vi "Config 135 via GPIB.vi"(3 "error in":T1, 4 "Configuration (in)":T3={"Sensor Length (cm)"=100.0, "Hi Setpoint (cm)"=80.0, "Lo Setpoint (cm)"=20.0, "Sampling Interval (min)"=1.0} {"Sampling Interval (min)" min=0 max=600 format="%.1f"; "Lo Setpoint (cm)" min=0 max=203.2 format="%.1f"; "Hi Setpoint (cm)" min=0 max=203.2 format="%.1f"; "Sensor Length (cm)" min=1 max=203.2 format="%.1f"}, 5 "Hidden Controls (in)":T2 {"Prev Sampling Interval" format="%.1f"; "Prev Lo Setpoint" format="%.1f"; "Prev Hi Setpoint" format="%.1f"; "Prev Sensor Length" format="%.1f"; "Helium Level (cm)" format="%.1f"}, 6 "GPIB Setup":cluster{"GPIB address":i16, "GPIB bus":i16}={"GPIB address"=1, "GPIB bus"=0}) -> (0 "error out":T1, 1 "Hidden Controls (out)":T2 {"Prev Sampling Interval" format="%.1f"; "Prev Lo Setpoint" format="%.1f"; "Prev Hi Setpoint" format="%.1f"; "Prev Sensor Length" format="%.1f"; "Helium Level (cm)" format="%.1f"}, 2 "Configuration (out)":T3={"Sensor Length (cm)"=100.0, "Hi Setpoint (cm)"=80.0, "Lo Setpoint (cm)"=20.0, "Sampling Interval (min)"=1.0} {"Sampling Interval (min)" min=0 max=600 format="%.1f"; "Lo Setpoint (cm)" min=0 max=203.2 format="%.1f"; "Hi Setpoint (cm)" min=0 max=203.2 format="%.1f"; "Sensor Length (cm)" min=1 max=203.2 format="%.1f"})   [LabVIEW 2016]
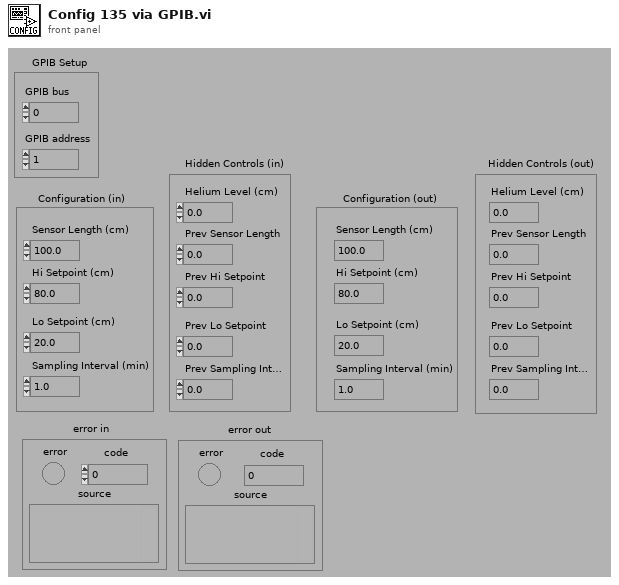
[diagram p1: front panel]
types:
  T1 = cluster{"error":bool, "code":i32, "source":string}
  T2 = cluster{"Helium Level (cm)":sgl, "Prev Sensor Length":sgl, "Prev Hi Setpoint":sgl, "Prev Lo Setpoint":sgl, "Prev Sampling Interval":sgl}
  T3 = cluster{"Sensor Length (cm)":sgl, "Hi Setpoint (cm)":sgl, "Lo Setpoint (cm)":sgl, "Sampling Interval (min)":sgl}
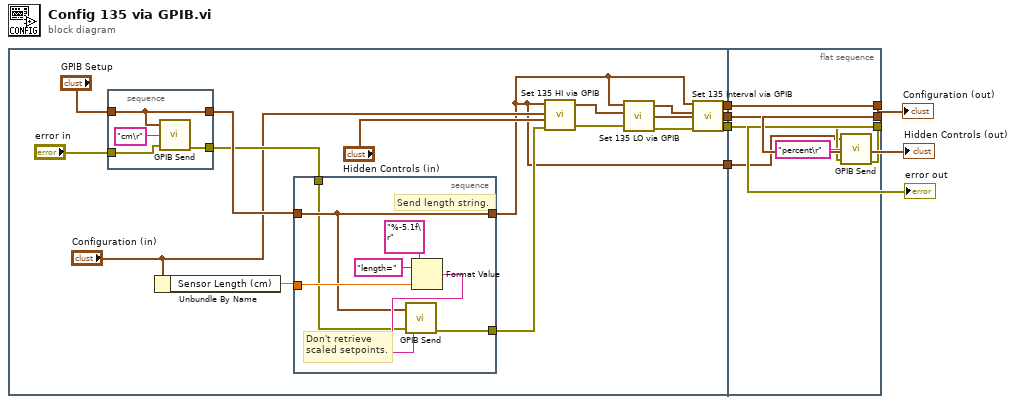
[diagram p0: block diagram]
diagram:
  n1 = flat-sequence {
    tunnel: [w21] -> w4
    tunnel: [w20] -> w3
    tunnel: [w13] -> w2
    tunnel: [w8] -> w1
    tunnel: [w38] -> w5
    tunnel: [w37] -> w6
    tunnel: [w41] -> w7
    tunnel: w4 -> [w41]
    tunnel: w3 -> [w37]
    tunnel: w2 -> [w39]
    tunnel: w1 -> [w36]
    frame #0 {
      n2 = stacked-sequence {
        tunnel: "GPIB Setup" -> [w35]
        tunnel: [w35] -> w23
        tunnel: [w34] -> w16
        tunnel: "error in" -> [w32]
        frame #0 {
          n3 = call "GPIB Send.vi"("GPIB Setup"=w35, "Input command"="cm\r", "error in"=w32) -> ("error out"=w34:T1)  [unwired: 3 out]
        }
      }
      n4 = Unbundle By Name("Configuration (in)") -> ("Sensor Length (cm)"=w22:sgl)
      n5 = stacked-sequence {
        tunnel: w22 -> [w30]
        tunnel: w23 -> [w27]
        tunnel: [w27] -> w8
        tunnel: w16 -> [w26]
        tunnel: [w25] -> w15
        frame #0 {
          # "Don't retrieve\nscaled setpoints."
          # "Send length string."
          n6 = Format Value(string ("")="length=", format string="%-5.1f\r", value (0)=w30) -> (output string=w31:string)
          n7 = call "GPIB Send.vi"("GPIB Setup"=w27, "Input command"=w31, "error in"=w26) -> ("error out"=w25:T1)  [unwired: 3 out]
        }
      }
      n8 = call "Set 135 HI via GPIB.vi"("error in"=w15, "Hidden Controls (in)"="Hidden Controls (in)", "Configuration (in)"="Configuration (in)", "GPIB Setup"=w8) -> ("error out"=w18:T1, "Configuration (out)"=w12:T3)  [unwired: 1 out]
      n9 = call "Set 135 LO via GPIB.vi"("error in"=w18, "Configuration (in)"=w12, "GPIB Setup"=w8) -> ("error out"=w17:T1, "Hidden Controls (out)"=w10:T2, "Configuration (out)"=w11:T3)  [unwired: 1 in]
      n10 = call "Set 135 Interval via GPIB.vi"("error in"=w17, "Hidden Controls (in)"=w10, "Configuration (in)"=w11, "GPIB Setup"=w8) -> ("error out"=w13:T1, "Hidden Controls (out)"=w20:T2, "Configuration (out)"=w21:T3)
    }
    frame #1 {
      n11 = call "GPIB Send.vi"("GPIB Setup"=w36, "Input command"="percent\r", "error in"=w39) -> ("error out"=w38:T1)  [unwired: 3 out]
    }
  }
  "Configuration (out)" <- w7
  "Hidden Controls (out)" <- w6
  "error out" <- w5
